vi "Heat_Tape_Global.vi"() -> ()   [LabVIEW 2019]
panel:
  out "HeatTape_T2":dbl
  out "HeatTape_ST":u32(colorbox)
  out "HeatTape_T1":dbl
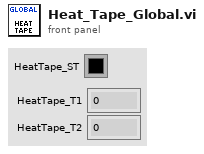
[diagram p1: front panel]
diagram:
